vi "StraightDrive.vi"(9 "RightDrive in":dbl, 10 "LeftDrive in":dbl, 11 "StraightDrive":bool) -> (1 "RightDrive out":dbl, 2 "LeftDrive out":dbl)   [LabVIEW 2013]
doc: "When StraightDrive is true, takes the left joystick value and makes that both the left and right joystick values. Otherwise, no action is taken."
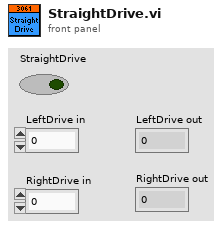
[diagram p1: front panel]
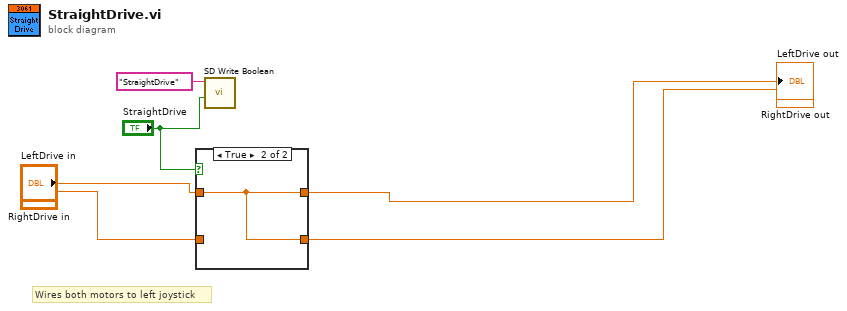
[diagram p0: block diagram]
diagram:
  # "Wires both motors to left joystick"
  n1 = case shown="True" "StraightDrive" {
    tunnel: [w8 w9] -> w5
    tunnel: "RightDrive in" -> [w8 _]
    tunnel: [w7 w9] -> w6
    tunnel: "LeftDrive in" -> [w7 w9]
    frame False {
    }
    frame True {
    }
  }
  "LeftDrive out" <- w6
  "RightDrive out" <- w5
  n2 = call <vilib>:"SD Write Boolean.vi"("Boolean"="StraightDrive", "Name"="StraightDrive") -> ()  [unwired: 8 in, 2 out]
